vi "setID.vi"(8 "error in (no error)":errorcluster, 10 "ID":u32, 11 "Node in":refnum<class "Node.lvclass">) -> (0 "error out":errorcluster, 3 "Node out":refnum<class "Node.lvclass">)   [LabVIEW 2009, in "Node.lvclass"]
uses:
  Node.lvclass
  Node.lvclass/Node.ctl
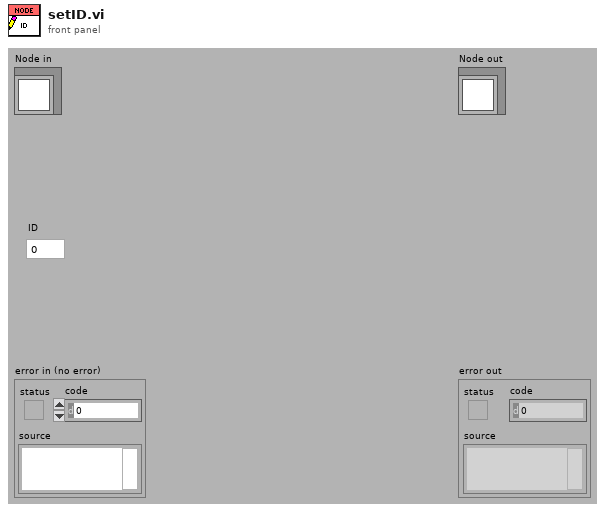
[diagram p1: front panel]
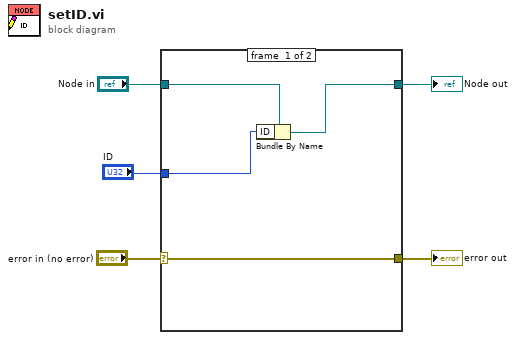
[diagram p0: block diagram]
diagram:
  n1 = case shown="No Error" "error in (no error)" {
    selector: "error in (no error)" -> [w6 w10]
    tunnel: [w6 w10] -> w4
    tunnel: [w7 w11] -> w2
    tunnel: "Node in" -> [w9 w11]
    tunnel: "ID" -> [w8 _]
    frame #0 {
      n2 = Bundle By Name(cluster=w9, "ID"=w8) -> (w7:refnum<class "Node.lvclass">)
    }
    frame #1 {
    }
  }
  "error out" <- w4
  "Node out" <- w2
